vi "读取名称.vi"(8 "error in (no error)":errorcluster caption="错误输入（无错误）", 11 "DATA输入":refnum<class "DATA.lvclass">) -> (0 "error out":errorcluster caption="错误输出", 2 "名称":string, 3 "DATA输出":refnum<class "DATA.lvclass">)   [LabVIEW 2011, in "List.lvlib" / "DATA.lvclass"]
uses:
  DATA.lvclass
  DATA.lvclass/DATA.ctl
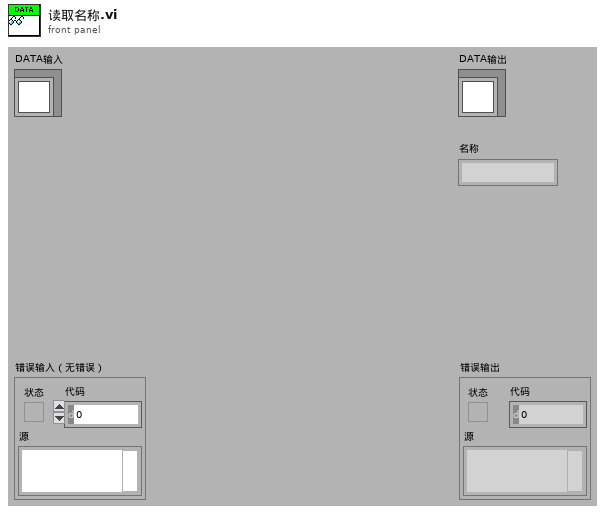
[diagram p1: front panel]
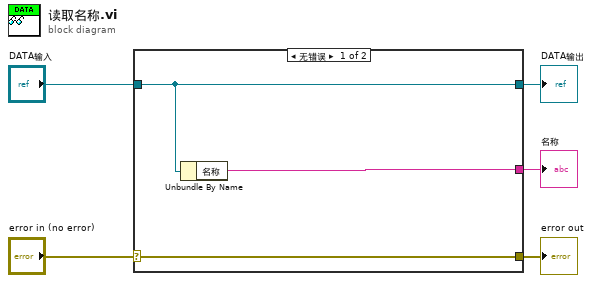
[diagram p0: block diagram]
diagram:
  n1 = case shown="无错误" "error in (no error)" {
    selector: "error in (no error)" -> [w8 w9]
    tunnel: [w8 w9] -> w4
    tunnel: [w7 w10] -> w2
    tunnel: "DATA输入" -> [w7 w10]
    tunnel: [w6 _] -> w1
    frame No Error {
      n2 = Unbundle By Name(w7) -> ("名称"=w6:string)
    }
    frame Error {
    }
  }
  "error out" <- w4
  "DATA输出" <- w2
  "名称" <- w1
